vi "WriteIOMerge.vi"   [LabVIEW 2020]
doc: "Writes new output data to the I/O items as soon as the target is ready to receive new data. This function does not overwrite previously written data."
uses:
  <vilib>/eio/EIOGrowableMethodNode/genericMethod/EIOGrowableMethodNode.xnode
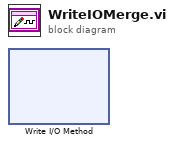
[diagram p0: block diagram]
diagram:
  n1 = xnode "Write I/O Method"() -> ()  [unwired: 3 in, 2 out]
